vi "Peroid Timer.vi"(1 "time(ms)":u32=1000, 2 "error in (no error)":errorcluster, 4 "Suspend?(F)":bool) -> (8 "time up?":bool=TRUE, 9 "error out":errorcluster)   [LabVIEW 2014]
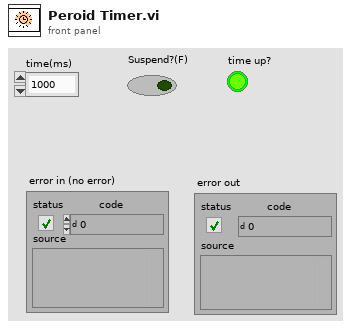
[diagram p1: front panel]
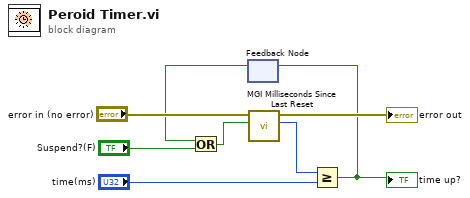
[diagram p0: block diagram]
diagram:
  n1 = feedback #1() -> (w2:bool)  [unwired: 1 in]
  n2 = Or(x=w2, y="Suspend?(F)") -> (x .or. y?=w1:bool)
  n3 = call <userlib>:"MGI Milliseconds Since Last Reset.vi"("Reset (F)"=w1, "Error In"="error in (no error)") -> ("ms"=w6:u32, "Error Out"=→"error out":errorcluster)  [unwired: 4 in]
  n4 = Greater Or Equal?(x=w6, y="time(ms)") -> (x >= y?=w4:bool)
  "time up?" <- w4
  n5 = feedback-in #1(w4) -> ()
